vi "Remove Subscription.vi"(8 "error in (no error)":errorcluster, 10 "Topic Filter":string, 11 "Client ID":string) -> (0 "error out":errorcluster)   [LabVIEW 2013, in "MQTT Server.lvlib" / "StoredSessions.lvclass"]
uses:
  StoredSessions.lvclass
  Session State -- cluster.ctl
  <vilib>/LabVIEW Open Source Project/MQTT Control Packets/Control Packets/SUBSCRIBE/Topic Subscription -- cluster.ctl
  <vilib>/LabVIEW Open Source Project/MQTT Control Packets/Control Packets/ControlPacket/QualityOfService -- enum.ctl
  <vilib>/LabVIEW Open Source Project/MQTT Control Packets/Control Packets/ControlPacket/ControlPacket.lvclass
  <vilib>/LabVIEW Open Source Project/MQTT Control Packets/Control Packets/SUBSCRIBE/SUBSCRIBE.lvclass
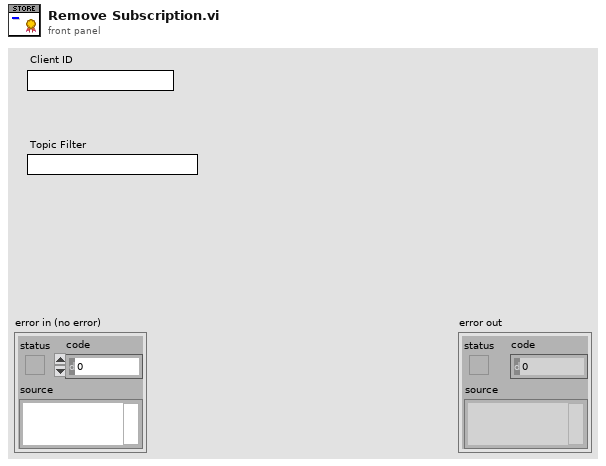
[diagram p1: front panel]
types:
  T1 = typedef "MQTT Server.lvlib/StoredSessions.lvclass/Session State -- cluster.ctl" = cluster{"Client ID":string, "Subscriptions":T2[], "PUBREC":u16[]}
  T2 = typedef "MQTT_Control_Packets.lvlib/SUBSCRIBE.lvclass/Topic Subscription -- cluster.ctl" = cluster{"Topic Filter":string, "QoS":T3}
  T3 = typedef "MQTT_Control_Packets.lvlib/ControlPacket.lvclass/QualityOfService -- enum.ctl" = enum16{"0 (At Most Once)", "1 (At Least Once)", "2 (Exactly Once)"}
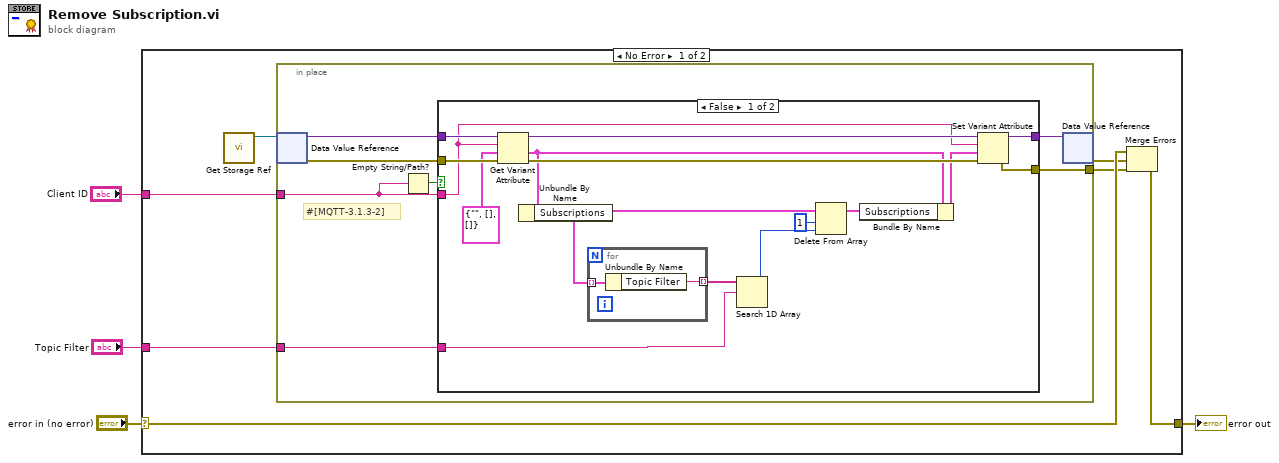
[diagram p0: block diagram]
diagram:
  n1 = case shown="No Error" "error in (no error)" {
    selector: "error in (no error)" -> [w11 w39]
    tunnel: [w10 w39] -> w3
    tunnel: "Topic Filter" -> [w9 _]
    tunnel: "Client ID" -> [w8 _]
    frame No Error {
      n2 = call "Get Storage Ref.vi"() -> ("Storage"=w7:refnum<data-value>)  [unwired: 11 in]
      n3 = in-place {
        in-place-border: w9 -> [w12]
        in-place-border: [w16] -> w5
        in-place-border: w8 -> [w13]
        # "#[MQTT-3.1.3-2]"
        n4 = in-place-dvr #1(w7) -> (w18:variant, w15:errorcluster)
        n5 = Empty String/Path?(string/path=w13) -> (empty?=w14:bool)
        n6 = case shown="False" w14 {
          tunnel: w18 -> [w34 w38]
          tunnel: [w31 w38] -> w17
          tunnel: [w20 w37] -> w16
          tunnel: w15 -> [w33 w37]
          tunnel: w13 -> [w28 _]
          tunnel: w12 -> [w19 _]
          frame False {
            n7 = Get Variant Attribute(Variant=w34, name=w28, default value (empty Variant)=T1 {"Client ID"="", "Subscriptions"=[], "PUBREC"=[]} ("Stored Session"), error in=w33) -> (duplicate Variant=w32:variant, value=w27:T1, error out=w29:errorcluster)  [unwired: 1 out]
            n8 = Unbundle By Name(w27) -> ("Subscriptions"=w23:T2[])
            n9 = for {
              tunnel: w23 -> [w36] mode=indexing
              tunnel: [w35] -> w25 mode=indexing
              n10 = Unbundle By Name(w36) -> ("Topic Filter"=w35:string)
            }
            n11 = Search 1D Array(1D array=w25, element=w19) -> (index of element=w22:i32)  [unwired: 1 in]
            n12 = Delete From Array(array=w23, length=1, index=w22) -> (array with subset deleted=w24:T2[])  [unwired: 1 out]
            n13 = Bundle By Name(cluster=w27, "Subscriptions"=w24) -> (w26:T1)
            n14 = Set Variant Attribute(Variant=w32, name=w28, value=w26, error in=w29) -> (Variant out=w31:variant, error out=w20:errorcluster)  [unwired: 1 out]
          }
          frame True {
          }
        }
        n15 = in-place-dvr #1(w17) -> (w6:errorcluster)  [unwired: 1 out]
      }
      n16 = Merge Errors(w11, w6, w5) -> (w10:errorcluster)
    }
    frame Error {
    }
  }
  "error out" <- w3
